vi "GA Get Ex Adc.vi"(6 "pClock":u32, 7 "nCount":i16, 8 "error in (no error)":errorcluster caption="错误输入（无错误）", 9 "pValue":i16, 10 "nADCNum":i16, 11 "nCardIndex":i16) -> (0 "error out":errorcluster caption="错误输出", 1 "pValue out":i16, 3 "function return":i32, 4 "pClock out":u32)   [LabVIEW 2015, in "GAS.lvlib"]
doc: "extern \"C\" __declspec(dllimport) int GA_GetExAdc(short nCardIndex,short nADCNum,short *pValue,short nCount=1,unsigned long *pClock=NULL);"
uses:
  <userlib>/BP_GAS/GAS.lvlib
  <userlib>/BP_GAS/GAS.dll
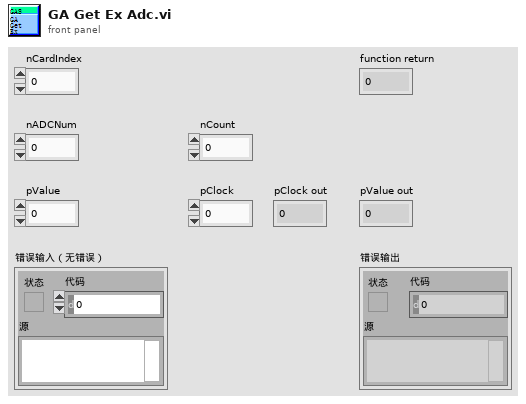
[diagram p1: front panel]
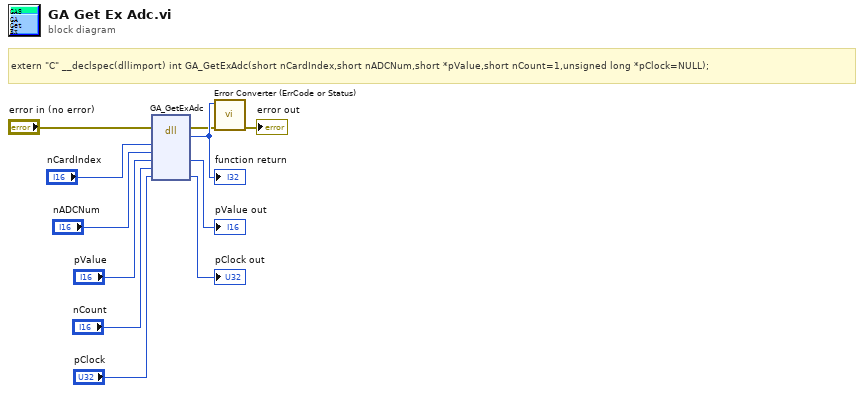
[diagram p0: block diagram]
diagram:
  # "extern \"C\" __declspec(dllimport) int GA_GetExAdc(short nCardIndex,short nADCNum,short *pValue,short nCount=1,unsigned long *pClock=NULL);"
  n1 = dll-call lib="E:/Program Files (x86)/National Instruments/LabVIEW 2015/user.lib/BP_GAS/GAS.*" fn="GA_GetExAdc"(error in="error in (no error)", "nCardIndex"="nCardIndex", "nADCNum"="nADCNum", "pValue"="pValue", "nCount"="nCount", "pClock"="pClock") -> (error out=w2:errorcluster, w11:i32, "pValue"=→"pValue out":i16, "pClock"=→"pClock out":u32)  [unwired: 5 in, 1 out]
  "function return" <- w11
  n2 = call "Error Converter (ErrCode or Status).vi"("error in (no error)"=w2, "error code"=w11) -> ("error out"=→"error out":errorcluster)  [unwired: 9 in]
